vi "TransAngle-180To180.vi"(1 "Angle":dbl) -> (0 "数值":dbl)   [LabVIEW 2014]
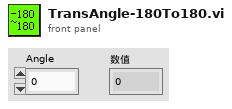
[diagram p1: front panel]
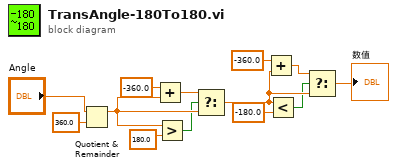
[diagram p0: block diagram]
diagram:
  n1 = Quotient & Remainder(x="Angle", y=360.0) -> (x-y*floor(x/y)=w13:dbl)  [unwired: 1 out]
  n2 = Add(x=-360.0, y=w13) -> (x+y=w4:dbl)
  n3 = Greater?(x=w13, y=180.0) -> (0:w2:bool)
  n4 = Select(t=w4, s=w2, f=w13) -> (s? t:f=w8:dbl)
  n5 = Add(x=-360.0, y=w8) -> (x+y=w9:dbl)
  n6 = Less?(x=w8, y=-180.0) -> (x < y?=w6:bool)
  n7 = Select(t=w9, s=w6, f=w8) -> (s? t:f=→"数值":dbl)
